vi "Pixel 2 Condition (SubVI).vi"(10 "Contour Scan in":T1, 11 "Fnd?":bool) -> (2 "Contour Scan out":T1)   [LabVIEW 2015]
uses:
  Controls (FPGA)/Contour Scan.ctl
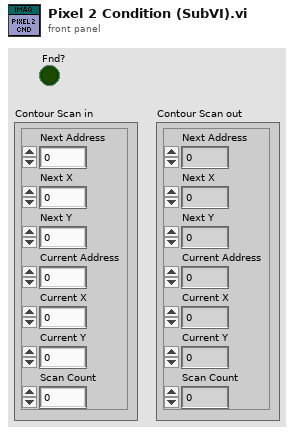
[diagram p1: front panel]
types:
  T1 = typedef "Contour Scan.ctl" = cluster{"Next Address":fxp<+,24,24>, "Next X":fxp<+,12,12>, "Next Y":fxp<+,12,12>, "Current Address":fxp<+,24,24>, "Current X":fxp<+,12,12>, "Current Y":fxp<+,12,12>, "Scan Count":u32}
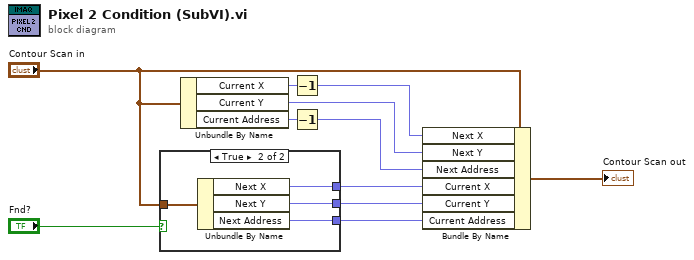
[diagram p0: block diagram]
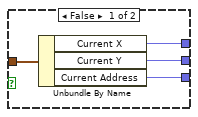
[diagram p2: hidden frame]
diagram:
  n1 = case shown="True" "Fnd?" {
    tunnel: "Contour Scan in" -> [w15 w19]
    tunnel: [w14 w18] -> w9
    tunnel: [w13 w17] -> w10
    tunnel: [w12 w16] -> w11
    frame False {
      n2 = Unbundle By Name(w15) -> ("Current X"=w14:fxp<+,12,12>, "Current Y"=w13:fxp<+,12,12>, "Current Address"=w12:fxp<+,24,24>)
    }
    frame True {
      n3 = Unbundle By Name(w19) -> ("Next X"=w18:fxp<+,12,12>, "Next Y"=w17:fxp<+,12,12>, "Next Address"=w16:fxp<+,24,24>)
    }
  }
  n4 = Unbundle By Name("Contour Scan in") -> ("Current X"=w5:fxp<+,12,12>, "Current Y"=w4:fxp<+,12,12>, "Current Address"=w2:fxp<+,24,24>)
  n5 = Decrement(x=w5) -> (x-1=w6:fxp<+,12,12>)
  n6 = Decrement(x=w2) -> (x-1=w3:fxp<+,24,24>)
  n7 = Bundle By Name(cluster="Contour Scan in", "Next X"=w6, "Next Y"=w4, "Next Address"=w3, "Current X"=w9, "Current Y"=w10, "Current Address"=w11) -> (→"Contour Scan out":T1)
